vi "CB Flywheel Model to PID.vi"(9 "control range (V)":cluster{dbl, dbl}, 10 "K (gain matrix)":T1, 11 "State Space Model":T2) -> (1 "feedforward":dbl, 2 "output range":cluster{dbl, dbl}, 3 "PID gains":cluster{"Real Matrix Element":dbl, dbl, dbl})   [LabVIEW 2020]
uses:
  CB State Space.ctl
  <vilib>/Analysis/Matrix/Datatypes/RealMatrix.ctl
  <vilib>/Analysis/Matrix/NI_Matrix.lvlib
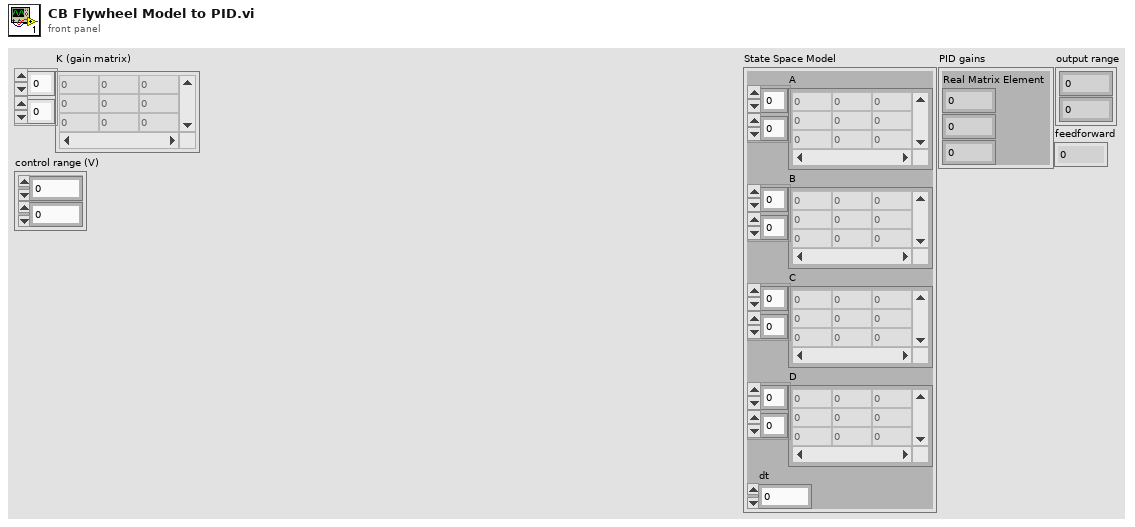
[diagram p1: front panel]
types:
  T1 = typedef "NI_Matrix.lvlib/RealMatrix.ctl" = dbl[][]
  T2 = typedef "CB State Space.ctl" = cluster{"A":T1, "B":T1, "C":T1, "D":T1, "dt":dbl}
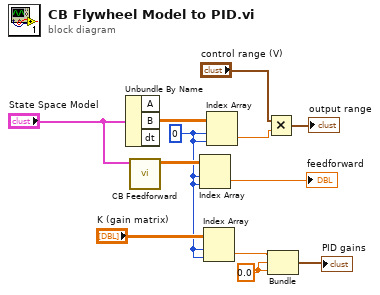
[diagram p0: block diagram]
diagram:
  w1 = 0 ("index (row)")
  w10 = 0.0
  n1 = Unbundle By Name("State Space Model") -> ("B"=w8:T1)  [unwired: 2 out]
  n2 = call "CB Feedforward.vi"("State Space Model"="State Space Model") -> ("Feed Forward"=w4:T1)  [unwired: 10 in]
  n3 = Index Array(array=w4, index (row)=w1, index (col)=w1) -> (element=→"feedforward":dbl)
  n4 = Index Array(array="K (gain matrix)", index (row)=w1, index (col)=w1) -> (element=w11:dbl)
  n5 = Index Array(array=w8, index (row)=w1, index (col)=w1) -> (element=w3:dbl)
  n6 = Multiply(x="control range (V)", y=w3) -> (x*y=→"output range":cluster{dbl, dbl})
  n7 = Bundle("Real Matrix Element"=w11, w10, w10) -> (→"PID gains":cluster{"Real Matrix Element":dbl, dbl, dbl})  [unwired: 1 in]
